vi "AlignTimeSeries.vi"(11 "time series in":T1[](array[typedef])) -> (3 "time series out":T1[](array[typedef]))   [LabVIEW 2017, in "TestPanel.lvlib"]
uses:
  <vilib>/addons/InsightCM/Devices/Shared/Common/TestPanel/TestPanel.lvlib
  <vilib>/addons/InsightCM/MessageBus/Base/controls/TestPanelTimeSeries.ctl
  <vilib>/addons/InsightCM/MessageBus/Base/controls/TestPanelValue.ctl
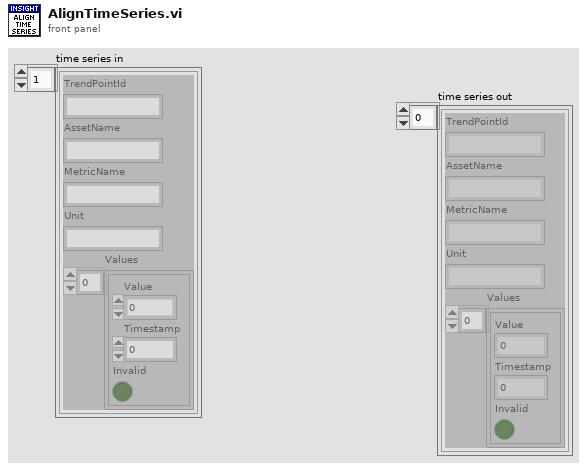
[diagram p1: front panel]
types:
  T1 = typedef "TestPanelTimeSeries.ctl" = cluster{"TrendPointId":string, "AssetName":string, "MetricName":string, "Unit":string, "Values":T2[]}
  T2 = typedef "TestPanelValue.ctl" = cluster{"Value":dbl, "Timestamp":i64, "Invalid":bool}
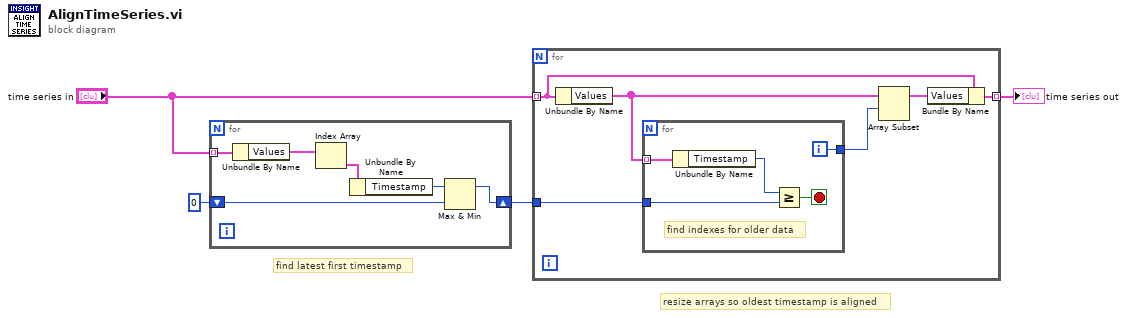
[diagram p0: block diagram]
diagram:
  # "resize arrays so oldest timestamp is aligned"
  # "find latest first timestamp"
  n1 = for {
    tunnel: "time series in" -> [w10] mode=indexing
    shift-right: [w5] -> w3
    shift-left: i64 0 -> [w6]
    n2 = Unbundle By Name(w10) -> ("Values"=w9:T2[])
    n3 = Index Array(array=w9) -> (element=w8:T2)  [unwired: 1 in]
    n4 = Unbundle By Name(w8) -> ("Timestamp"=w7:i64)
    n5 = Max & Min(x=w7, y=w6) -> (max(x,y)=w5:i64)  [unwired: 1 out]
  }
  n6 = for {
    tunnel: "time series in" -> [w13] mode=indexing
    tunnel: w3 -> [w16]
    tunnel: [w11] -> w1 mode=indexing
    n7 = Unbundle By Name(w13) -> ("Values"=w15:T2[])
    n8 = for {
      tunnel: w15 -> [w21] mode=indexing
      tunnel: w16 -> [w19]
      tunnel: [w17] -> w14
      i -> [w17]
      stop <- w18 stop-if-true
      # "find indexes for older data"
      n9 = Unbundle By Name(w21) -> ("Timestamp"=w20:i64)
      n10 = Greater Or Equal?(x=w20, y=w19) -> (x >= y?=w18:bool)
    }
    n11 = Array Subset(array=w15, index=w14) -> (w12:T2[])  [unwired: 1 in]
    n12 = Bundle By Name(cluster=w13, "Values"=w12) -> (w11:T1)
  }
  "time series out" <- w1
